vi "get one frame - subvi.vi"(8 "error in":errorcluster, 9 "Image Height":i32, 10 "Image Width":i32, 11 "Image In":T1) -> (0 "error out":errorcluster, 3 "Image Out":T1)   [LabVIEW 2014]
uses:
  <vilib>/vision/Image Controls.llb/IMAQ Image.ctl
  lib/Andorlib/atmcd32d.lvlib
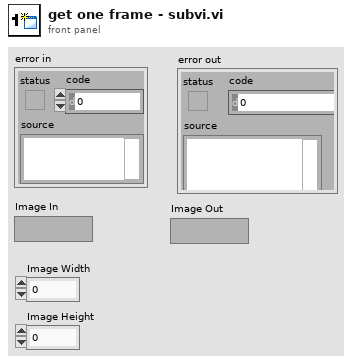
[diagram p1: front panel]
types:
  T1 = typedef "IMAQ Image.ctl" = refnum<image>
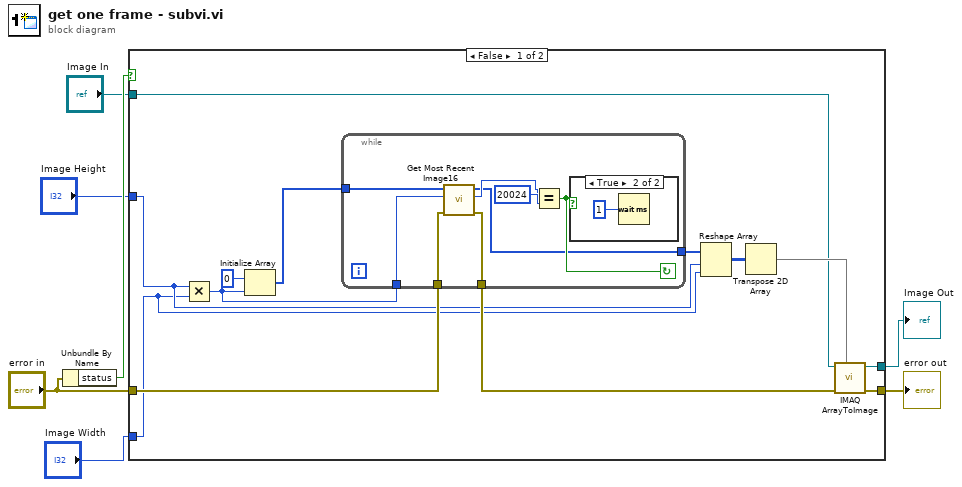
[diagram p0: block diagram]
diagram:
  n1 = Unbundle By Name("error in") -> ("status"=w7:bool)
  n2 = case shown="False" w7 {
    tunnel: "error in" -> [w16 w31]
    tunnel: [w20 w31] -> w2
    tunnel: "Image Height" -> [w11 _]
    tunnel: "Image Width" -> [w10 _]
    tunnel: "Image In" -> [w8 w30]
    tunnel: [w19 w30] -> w1
    frame False {
      n3 = Multiply(x=w11, y=w10) -> (x*y=w13:i32)
      n4 = Initialize Array(u16 0, w13) -> (w14:u16[])
      n5 = while {
        tunnel: [w28] -> w17
        tunnel: w16 -> [w24]
        tunnel: w14 -> [w23]
        tunnel: w13 -> [w22]
        tunnel: [w21] -> w12
        stop <- w25 continue-if-true
        n6 = call "Get Most Recent Image16.vi"("error in (no error)"=w24, "size"=w22, "Array 2"=w23) -> ("error out"=w28:errorcluster, "function return"=w26:u32, "Array"=w21:u16[])  [unwired: 6 in]
        n7 = Equal?(x=w26, y=20024) -> (x = y?=w25:bool)
        n8 = case shown="True" w25 {
          frame False {
          }
          frame True {
            n9 = Wait (ms)(milliseconds to wait=u32 1) -> ()  [unwired: 1 out]
          }
        }
      }
      n10 = Reshape Array(w12, w11, w10) -> (w18:u16[][])
      n11 = Transpose 2D Array(2D array=w18) -> (transposed array=w9:u16[][])
      n12 = call "IMAQ ArrayToImage"("Image Pixels (U16)"=w9, "error in (no error)"=w17, "Image"=w8) -> ("error out"=w20:errorcluster, "Image Out"=w19:T1)  [unwired: 3 in, 4 out]
    }
    frame True {
    }
  }
  "error out" <- w2
  "Image Out" <- w1
